vi "FPGA(test)_.vi"() -> ()   [LabVIEW 2019]
uses:
  <vilib>/rvi/Emulation/niFpgaGetClockAttributes.vi
  <vilib>/rvi/Emulation/niFpgaSctlEmulationGetInTimedLoop.vi
  <vilib>/rvi/Emulation/niFpgaEmulationReportErrorSimple.vi
  <vilib>/rvi/Emulation/niFpgaProcessEmulError.vi
  <vilib>/rvi/eio/common/nirviEmuTemplateMethod_errors.vi
  <vilib>/rvi/Emulation/niFpgaCriticalErrorInLSC.vi
  <vilib>/eio/EIONode/EIONode.xnode
panel:
  out "pwm_out":i32
  in  "angle_DIR":bool
  in  "pwm input(escon)":i32
  in  "Enable (escon)":bool
  in  "T(escon)":i32=20000
  out "Encoder  (4x)":i32
  out "Encoder  (1x)":i32
  in  "encoder reset":bool
  out "Encoder  (2x)":i32
  in  "stop":bool
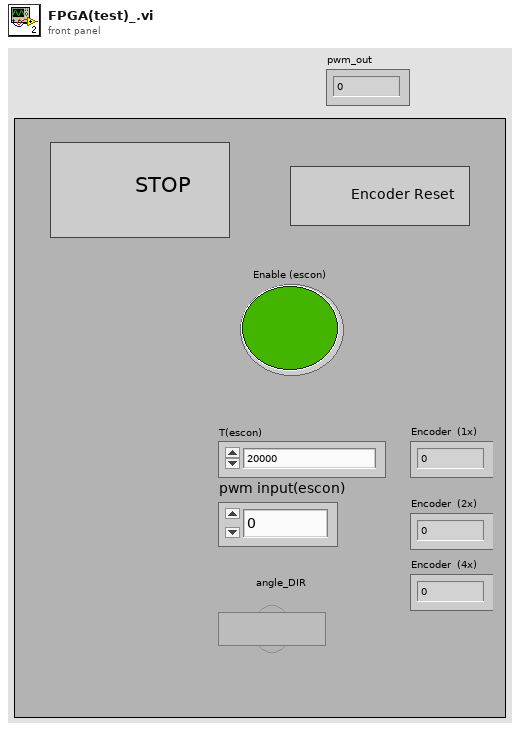
[diagram p1: front panel]
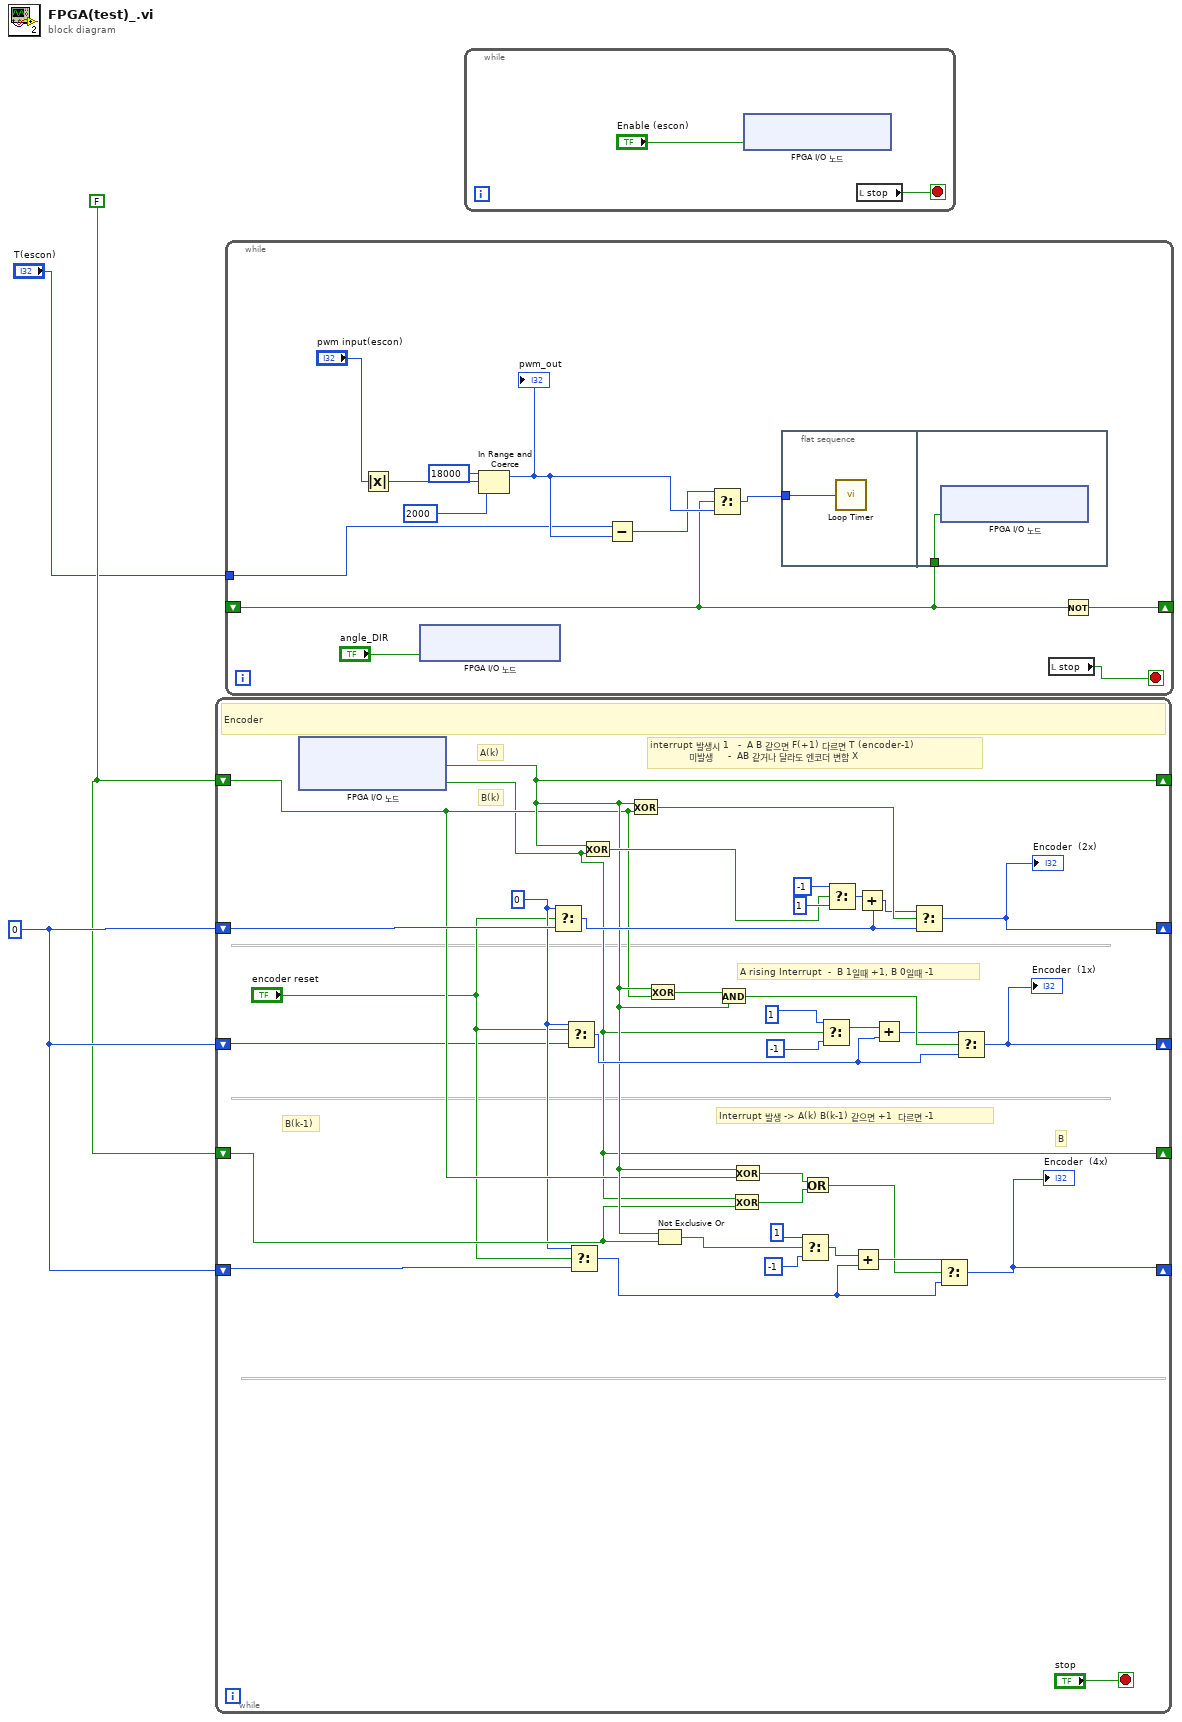
[diagram p0: block diagram]
diagram:
  w3 = 0
  w2 = FALSE
  n1 = while {
    shift-right: [w16] -> _
    shift-left: w2 -> [w15]
    shift-right: [w11] -> _
    shift-left: w3 -> [w35]
    shift-right: [w14] -> _
    shift-left: w2 -> [w13]
    shift-right: [w7] -> _
    shift-left: w3 -> [w6]
    shift-right: [w5] -> _
    shift-left: w3 -> [w4]
    stop <- "stop" stop-if-true
    w9 = 0 ("t")
    # "B"
    # "B(k-1)"
    # "Interrupt 발생 -> A(k) B(k-1) 같으면 +1  다르면 -1"
    # "A rising Interrupt  -  B 1일때 +1, B 0일때 -1"
    # "B(k)"
    # "A(k)"
    # "interrupt 발생시 1   -  A B 같으면 F(+1) 다르면 T (encoder-1)\n             미발생     -  AB 같거나 달라도 엔코더 변함 X"
    # "Encoder"
    n2 = xnode "FPGA I/O 노드"() -> ("ConnectorA/DIO9"=w16:bool, "ConnectorA/DIO10"=w14:bool)  [unwired: 2 in, 2 out]
    n3 = Select(t=w9, s="encoder reset", f=w35) -> (s? t:f=w34:i32)
    n4 = Select(t=w9, s="encoder reset", f=w6) -> (s? t:f=w27:i32)
    n5 = Select(t=w9, s="encoder reset", f=w4) -> (s? t:f=w10:i32)
    n6 = Exclusive Or(1:w14, 2:w16) -> (0:w26:bool)
    n7 = Exclusive Or(1:w15, 2:w16) -> (0:w39:bool)
    n8 = Exclusive Or(1:w15, 2:w16) -> (0:w33:bool)
    n9 = Not Exclusive Or(1:w13, 2:w16) -> (0:w22:bool)
    n10 = And(x=w33, y=w16) -> (x .and. y?=w32:bool)
    n11 = Exclusive Or(1:w13, 2:w14) -> (0:w18:bool)
    n12 = Exclusive Or(1:w15, 2:w16) -> (0:w19:bool)
    n13 = Select(t=i16 1, s=w22, f=i16 -1) -> (s? t:f=w21:i16)
    n14 = Or(x=w19, y=w18) -> (x .or. y?=w17:bool)
    n15 = Select(t=i16 1, s=w14, f=i16 -1) -> (s? t:f=w30:i16)
    n16 = Select(t=i16 -1, s=w26, f=i16 1) -> (s? t:f=w38:i16)
    n17 = Add(x=w21, y=w10) -> (x+y=w20:i32)
    n18 = Add(x=w38, y=w34) -> (x+y=w37:i32)
    n19 = Add(x=w30, y=w27) -> (x+y=w31:i32)
    n20 = Select(t=w37, s=w39, f=w34) -> (s? t:f=w11:i32)
    "Encoder  (2x)" <- w11
    n21 = Select(t=w20, s=w17, f=w10) -> (s? t:f=w5:i32)
    "Encoder  (4x)" <- w5
    n22 = Select(t=w31, s=w32, f=w27) -> (s? t:f=w7:i32)
    "Encoder  (1x)" <- w7
  }
  n23 = while {
    shift-right: [w46] -> _
    shift-left: _ -> [w45]
    tunnel: "T(escon)" -> [w44]
    stop <- w41 stop-if-true
    n24 = Absolute Value(x="pwm input(escon)") -> (abs(x)=w51:i32)
    n25 = xnode "FPGA I/O 노드"("ConnectorA/DIO8"="angle_DIR") -> ()  [unwired: 1 in, 1 out]
    n26 = In Range and Coerce(upper limit=i16 18000, x=w51, lower limit=i16 2000) -> (coerced(x)=w49:i32)  [unwired: 1 out]
    "pwm_out" <- w49
    n27 = Subtract(x=w44, y=w49) -> (x-y=w48:i32)
    n28 = Select(t=w48, s=w45, f=w49) -> (s? t:f=w47:i32)
    n29 = flat-sequence {
      tunnel: w47 -> [w52]
      tunnel: w45 -> [w53]
      frame #0 {
        n30 = call "Loop Timer"("Count(Ticks)"=w52) -> ()  [unwired: 1 out]
      }
      frame #1 {
        n31 = xnode "FPGA I/O 노드"("ConnectorA/DIO14"=w53) -> ()  [unwired: 1 in, 1 out]
      }
    }
    n32 = local read "stop"() -> (w41:bool)
    n33 = Not(x=w45) -> (.not. x?=w46:bool)
  }
  n34 = while {
    stop <- w54 stop-if-true
    n35 = xnode "FPGA I/O 노드"("ConnectorA/DIO15"="Enable (escon)") -> ()  [unwired: 1 in, 1 out]
    n36 = local read "stop"() -> (w54:bool)
  }
